vi "TestStand_Control ( Keyword_TestCase_Linkage ).vi"(11 "Test_Case":string="\nPrecondition:\nPC_1. Wait.Sec(Delay=2) // Wait for Sec\n\nTestProcedure:\nTP_1. Wait.mSec(Delay=1000)  //Waits for ms\n\nReset:\nRST_1. Wait.Sec(Delay=2)  //Waits for sec\r\n") -> (1 "Reset":T1[](array[typedef]), 2 "TestProcedure":T1[](array[typedef]), 3 "PreCondition":T1[](array[typedef]))   [LabVIEW 2018, in "TestStand_Control.lvlib"]
uses:
  TestStand_Control.lvlib
  Module_Controls/TestStand ( KWD_Info ).ctl
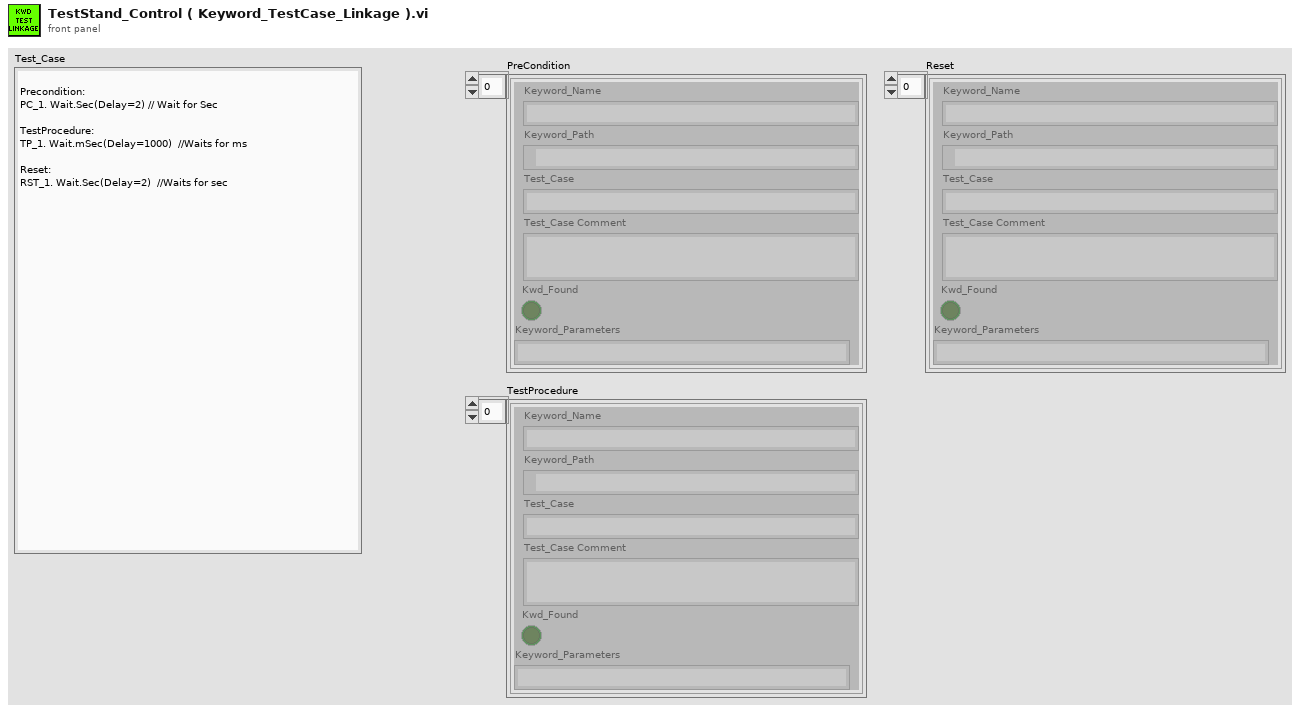
[diagram p1: front panel]
types:
  T1 = typedef "TestStand ( KWD_Info ).ctl" = cluster{"Keyword_Name":string, "Keyword_Path":path, "Test_Case":string, "Test_Case Comment":string, "Kwd_Found":bool, "Keyword_Parameters":string}
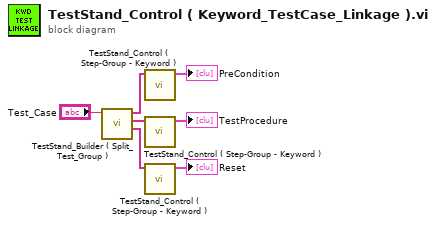
[diagram p0: block diagram]
diagram:
  n1 = call "TestStand_Builder ( Split_Test_Group ).vi"("Test_Case"="Test_Case") -> ("Reset"=w3:string[], "TestProcedure"=w4:string[], "Preconditions"=w6:string[])  [unwired: 8 in]
  n2 = call "TestStand_Control ( Step-Group - Keyword ).vi"("Step_group"=w6) -> ("Array"=→"PreCondition":T1[])  [unwired: 10 in]
  n3 = call "TestStand_Control ( Step-Group - Keyword ).vi"("Step_group"=w4) -> ("Array"=→"TestProcedure":T1[])  [unwired: 10 in]
  n4 = call "TestStand_Control ( Step-Group - Keyword ).vi"("Step_group"=w3) -> ("Array"=→"Reset":T1[])  [unwired: 10 in]
